vi "CalculateGroupPhasors.vi"(8 "error in":errorcluster, 10 "current waveforms":waveform(dbl)[](array[waveform]), 11 "phase voltage waveforms":waveform(dbl)[](array[waveform])) -> (0 "error out":errorcluster, 3 "Group Voltage Phasors":T1[](array[typedef]))   [LabVIEW 2017, in "McsaAnalysisLowRate.lvlib"]
uses:
  <vilib>/addons/InsightCM/Devices/Shared/Mcsa/McsaAnalysisLowRate/McsaAnalysisLowRate.lvlib
  <vilib>/addons/InsightCM/Utilities/Analysis/MCSA/controls/McsaChannelPhasor.ctl
  <vilib>/Analysis/coordinate.llb/Angle Range (Degree).ctl
  <vilib>/Analysis/coordinate.llb/Angle Units.ctl
  <vilib>/Analysis/coordinate.llb/Wrap Angle (scalar).vi
  <vilib>/addons/Electrical Power/Basic/Measurement/Fundamental Vector (N Channels).vi
  <vilib>/addons/Electrical Power/Basic/NI_EP_Basic.lvlib
  <vilib>/Analysis/NI_AAL_Angle.lvlib
  <vilib>/Analysis/NI_AALPro.lvlib
  <vilib>/addons/InsightCM/Utilities/Analysis/MCSA/McsaAnalysisFunctions.lvlib
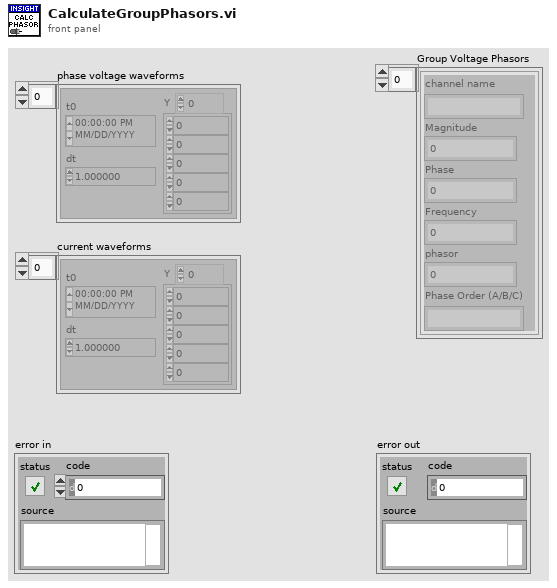
[diagram p1: front panel]
types:
  T1 = typedef "McsaAnalysisFunctions.lvlib/McsaChannelPhasor.ctl" = cluster{"channel name":string, "Magnitude":dbl, "Phase":dbl, "Frequency":dbl, "phasor":cdb, "Phase Order (A/B/C)":string}
  T2 = typedef "NI_AAL_Angle.lvlib/Angle Units.ctl" = i32
  T3 = typedef "NI_AAL_Angle.lvlib/Angle Range (Degree).ctl" = u16
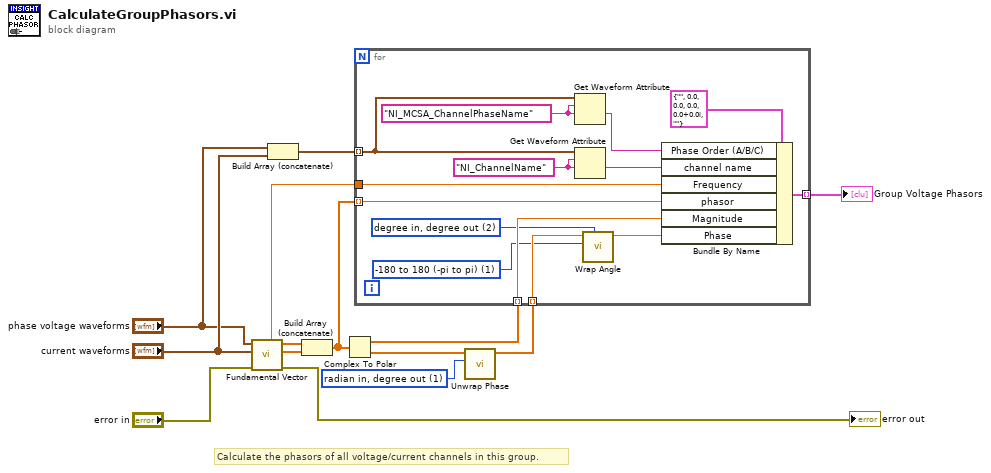
[diagram p0: block diagram]
diagram:
  w9 = 1 items=["radian in, radian out", "radian in, degree out", "degree in, degree out", "degree in, radian out"] ("phase unit")
  # "Calculate the phasors of all voltage/current channels in this group."
  n1 = call-poly <vilib>:"Fundamental Vector.vi"("error in (no error)"="error in", "current waveforms"="current waveforms", "voltage waveforms"="phase voltage waveforms") -> ("error out"=→"error out":errorcluster, "current fundamental vectors"=w12:cdb[], "voltage fundamental vectors"=w13:cdb[], "frequency"=w14:dbl)  [unwired: 5 in]
  n2 = Build Array (concatenate)("phase voltage waveforms", "current waveforms") -> (w10:waveform(dbl)[])
  n3 = Build Array (concatenate)(w13, w12) -> (w3:cdb[])
  n4 = Complex To Polar(r * e^(i*theta)=w3) -> (r=w7:dbl[], theta=w8:dbl[])
  n5 = call <vilib>:"Unwrap Phase.vi"("phase unit"=w9, "Phase"=w8) -> ("Unwrapped Phase"=w6:dbl[])  [unwired: 8 in, 1 out]
  n6 = for {
    tunnel: w10 -> [w21] mode=indexing
    tunnel: w14 -> [w26]
    tunnel: w7 -> [w23] mode=indexing
    tunnel: w6 -> [w18] mode=indexing
    tunnel: [w25] -> w1 mode=indexing
    tunnel: w3 -> [w22] mode=indexing
    w15 = T2 2 items=["radian in, radian out", "radian in, degree out", "degree in, degree out", "degree in, radian out"] ("angle units")
    w16 = T3 1 items=["none", "-180 to 180 (-pi to pi)", "0 to 360 (0 to 2pi)"] ("angle range")
    w20 = "NI_MCSA_ChannelPhaseName" ("name")
    w28 = "NI_ChannelName" ("name")
    n7 = Get Waveform Attribute(5:w20, 6:w20, 7:w21) -> (1:w19:string)  [unwired: 1 in, 3 out]
    n8 = Get Waveform Attribute(5:w28, 6:w28, 7:w21) -> (1:w24:string)  [unwired: 1 in, 3 out]
    n9 = call-poly <vilib>:"Wrap Angle.vi"("angle units"=w15, "angle range"=w16, "angle in"=w18) -> ("angle out"=w17:dbl)  [unwired: 7 in, 1 out]
    n10 = Bundle By Name(cluster=T1 {"channel name"="", "Magnitude"=0.0, "Phase"=0.0, "Frequency"=0.0, "phasor"=0.0+0.0i, "Phase Order (A/B/C)"=""} ("Channel Phasor"), "Phase Order (A/B/C)"=w19, "channel name"=w24, "Frequency"=w26, "phasor"=w22, "Magnitude"=w23, "Phase"=w17) -> (w25:T1)
  }
  "Group Voltage Phasors" <- w1
